vi "ModuleName.vi"(9 "Name":string="Module", 10 "ModuleID":i32=-1) -> (2 "ModuleName":string)   [LabVIEW 2018, in "ModuleAdmin.lvlib" / "ModuleAdmin.lvclass"]
doc: "Creates a module name by combining the name and ModuleID."
uses:
  ModuleAdmin.lvclass
panel:
  out "Error Out":errorcluster
  in  "Error In":errorcluster
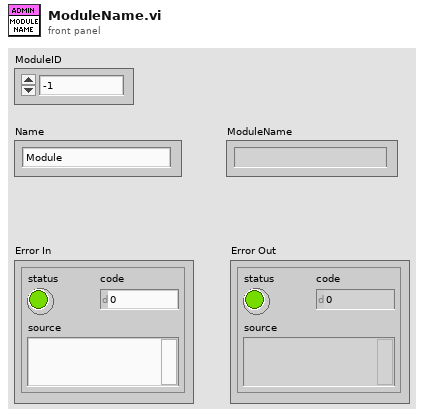
[diagram p1: front panel]
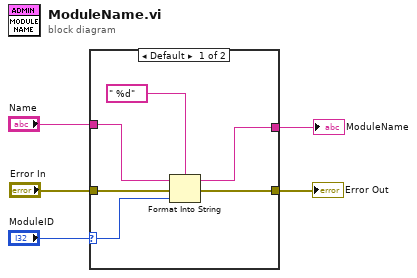
[diagram p0: block diagram]
diagram:
  n1 = case shown="Default" "ModuleID" {
    selector: "ModuleID" -> [w11 _]
    tunnel: [w9 w13] -> w3
    tunnel: "Name" -> [w10 w13]
    tunnel: [w7 w12] -> w2
    tunnel: "Error In" -> [w6 w12]
    frame Default {
      n2 = Format Into String(format string=" %d", initial string=w10, error in=w6, w11) -> (resulting string=w9:string, error out=w7:errorcluster)
    }
    frame ..-1 {
    }
  }
  "ModuleName" <- w3
  "Error Out" <- w2
